vi "Calculate Time to Achieve Slew Rate.vi"(9 "Current/voltage set point 2":dbl, 10 "Current/voltage set point 1":dbl, 11 "Current/voltage slew rate":dbl) -> (3 "Calculated time":dbl)   [LabVIEW 2021, in "PMIC Common.lvlib"]
uses:
  PMIC Common.lvlib
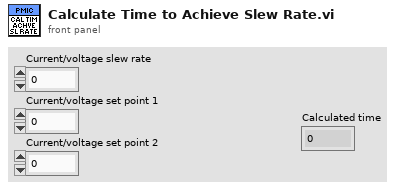
[diagram p1: front panel]
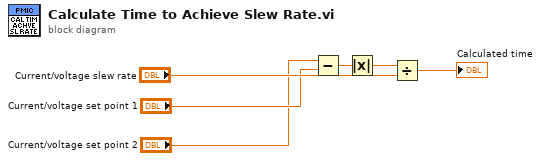
[diagram p0: block diagram]
diagram:
  n1 = Subtract(x="Current/voltage set point 2", y="Current/voltage set point 1") -> (x-y=w3:dbl)
  n2 = Absolute Value(x=w3) -> (abs(x)=w4:dbl)
  n3 = Divide(x=w4, y="Current/voltage slew rate") -> (x/y=→"Calculated time":dbl)
